vi "error_handler.vi"(9 "IC6 error code":string, 10 "Error type":T1(ring)) -> (0 "error out":errorcluster)   [LabVIEW 2018]
doc: "Handle errors read from a command response packet."
uses:
  <vilib>/Utility/error.llb/DialogType.ctl
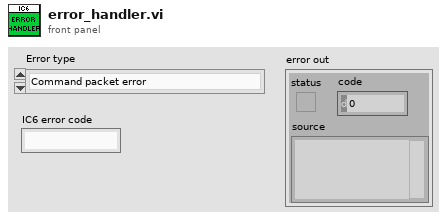
[diagram p1: front panel]
types:
  T1 = enum16{"Command packet error", "Checksum not verified", "Command not acknowledged"}
  T2 = typedef "DialogType.ctl" = u16
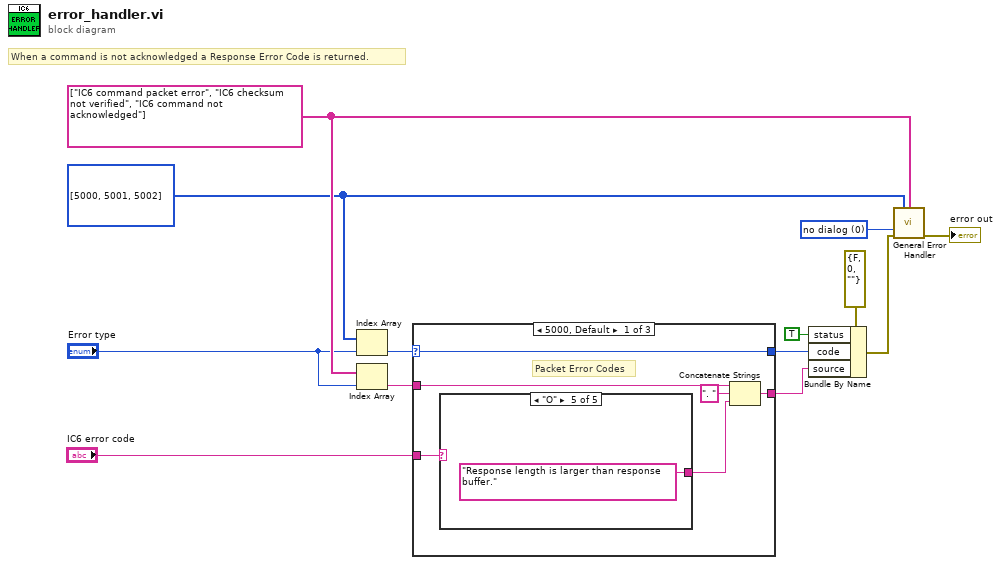
[diagram p0: block diagram]
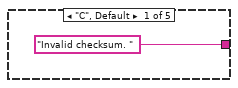
[diagram p2: hidden frame]
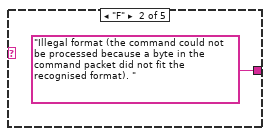
[diagram p3: hidden frame]
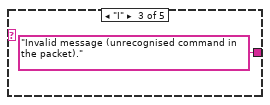
[diagram p4: hidden frame]
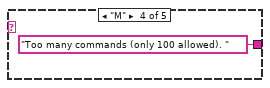
[diagram p5: hidden frame]
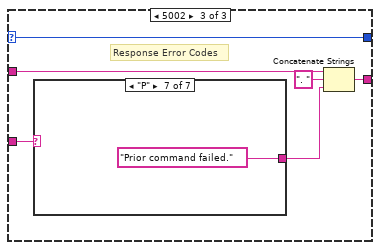
[diagram p7: hidden frame]
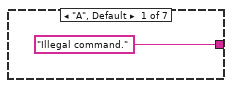
[diagram p8: hidden frame]
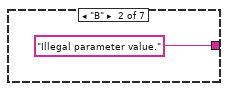
[diagram p9: hidden frame]
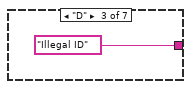
[diagram p10: hidden frame]
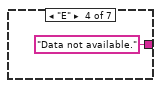
[diagram p11: hidden frame]
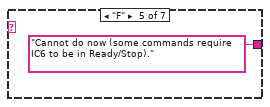
[diagram p12: hidden frame]
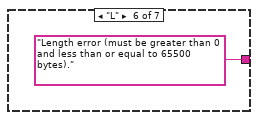
[diagram p13: hidden frame]
diagram:
  w12 = T2 0 items=["no dialog", "OK message", "continue or stop message", "OK message + warnings", "continue/stop + warnings"] ("type of dialog (OK msg:1)")
  w11 = string[] ["IC6 command packet error", "IC6 checksum not verified", "IC6 command not acknowledged"] ("[user-defined descriptions]")
  w7 = i32[] [5000, 5001, 5002] ("[user-defined codes]")
  # "When a command is not acknowledged a Response Error Code is returned."
  n1 = Index Array(array=w7, index="Error type") -> (element=w5:i32)
  n2 = Index Array(array=w11, index="Error type") -> (element=w2:string)
  n3 = case shown="5000, Default" w5 {
    selector: w5 -> [w16 w26 w32]
    tunnel: "IC6 error code" -> [w18 _ w29]
    tunnel: [w16 w26 w32] -> w3
    tunnel: w2 -> [w15 w25 w28]
    tunnel: [w14 w25 w27] -> w1
    frame 5000, Default {
      # "Packet Error Codes"
      n4 = case shown="\"O\"" w18 {
        tunnel: ["Invalid checksum. " ("string") "Illegal format (the command could not be processed because a byte in the command packet did not fit the recognised format). " ("string") "Invalid message (unrecognised command in the packet)." ("string") "Too many commands (only 100 allowed). " ("string") "Response length is larger than response buffer." ("string")] -> w17
        frame "C", Default {
        }
        frame "F" {
        }
        frame "I" {
        }
        frame "M" {
        }
        frame "O" {
        }
      }
      n5 = Concatenate Strings(w15, ". " ("string"), w17) -> (w14:string)
    }
    frame 5001 {
    }
    frame 5002 {
      # "Response Error Codes"
      n6 = case shown="\"P\"" w29 {
        tunnel: ["Illegal command." ("string") "Illegal parameter value." ("string") "Illegal ID" ("string") "Data not available." ("string") "Cannot do now (some commands require IC6 to be in Ready/Stop)." ("string") "Length error (must be greater than 0 and less than or equal to 65500 bytes)." ("string") "Prior command failed." ("string")] -> w31
        frame "A", Default {
        }
        frame "B" {
        }
        frame "D" {
        }
        frame "E" {
        }
        frame "F" {
        }
        frame "L" {
        }
        frame "P" {
        }
      }
      n7 = Concatenate Strings(w28, ". " ("string"), w31) -> (w27:string)
    }
  }
  n8 = Bundle By Name(cluster=errorcluster {"status"=FALSE, "code"=0, "source"=""} ("error out"), "status"=TRUE, "code"=w3, "source"=w1) -> (w6:errorcluster)
  n9 = call <vilib>:"General Error Handler.vi"("[user-defined codes]"=w7, "[user-defined descriptions]"=w11, "type of dialog (OK msg:1)"=w12, "error in (no error)"=w6) -> ("error out"=→"error out":errorcluster)  [unwired: 7 in, 4 out]
